vi "slide.vi"(11 "Slide in":refnum<vi>) -> ()   [LabVIEW 2016]
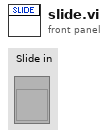
[diagram p1: front panel]
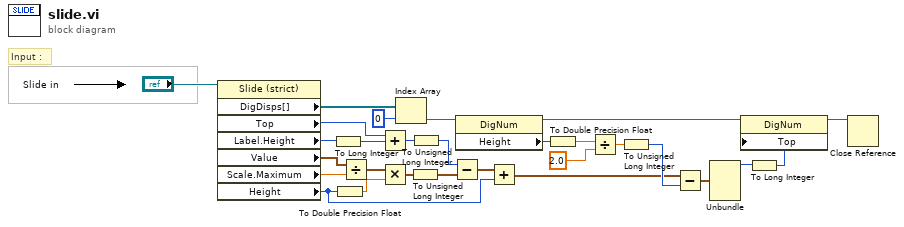
[diagram p0: block diagram]
diagram:
  # "Input :"
  n1 = property class="Slide (strict)"(reference="Slide in") -> ("DigDisps[]"=w27:refnum<vi>[], "Top"=w7:i32, "Label.Height"=w9:u32, "Value"=w17:cluster{dbl, dbl, dbl, dbl, dbl}, "Scale.Maximum"=w16:dbl, "Height"=w5:u32)  [unwired: 1 in, 2 out]
  n2 = To Long Integer(number=w9) -> (32bit integer=w8:i32)
  n3 = To Double Precision Float(number=w5) -> (double precision float=w6:dbl)
  n4 = Divide(x=w17, y=w16) -> (x/y=w15:cluster{dbl, dbl, dbl, dbl, dbl})
  n5 = Add(x=w7, y=w8) -> (x+y=w3:i32)
  n6 = Multiply(x=w15, y=w6) -> (x*y=w20:cluster{dbl, dbl, dbl, dbl, dbl})
  n7 = Index Array(array=w27, index=0) -> (element=w26:refnum<vi>)
  n8 = To Unsigned Long Integer(number=w20) -> (unsigned 32bit integer=w19:cluster{u32, u32, u32, u32, u32})
  n9 = To Unsigned Long Integer(number=w3) -> (unsigned 32bit integer=w4:u32)
  n10 = Subtract(x=w4, y=w19) -> (x-y=w18:cluster{u32, u32, u32, u32, u32})
  n11 = property class="DigNum"(reference=w26) -> (reference out=w24:refnum<vi>, "Height"=w12:u32)  [unwired: 1 in, 1 out]
  n12 = Add(x=w18, y=w5) -> (x+y=w10:cluster{u32, u32, u32, u32, u32})
  n13 = To Double Precision Float(number=w12) -> (double precision float=w11:dbl)
  n14 = Divide(x=w11, y=2.0) -> (x/y=w22:dbl)
  n15 = To Unsigned Long Integer(number=w22) -> (unsigned 32bit integer=w21:u32)
  n16 = Subtract(x=w10, y=w21) -> (x-y=w14:cluster{u32, u32, u32, u32, u32})
  n17 = Unbundle(w14) -> (w2:u32)  [unwired: 4 out]
  n18 = To Long Integer(number=w2) -> (32bit integer=w1:i32)
  n19 = property class="DigNum"(reference=w24, "Top"=w1) -> (reference out=w13:refnum<vi>)  [unwired: 1 in, 1 out]
  n20 = Close Reference(reference=w13) -> ()  [unwired: 1 in, 1 out]
